vi "ConvertControlTerminals.vi"(5 "PythonConverter_BD in":refnum<class "PyConvBD.lvclass">, 6 "error in":errorcluster, 9 "Diagram in":refnum<class "Diagram.lvclass">) -> (0 "error out":errorcluster, 3 "Diagram out":refnum<class "Diagram.lvclass">, 4 "PythonConverter_BD out":refnum<class "PyConvBD.lvclass">)   [LabVIEW 2014, in "Raspberry Pi Compatible Compiler for LabVIEW.lvlib" / "Diagram.lvclass"]
uses:
  Diagram.lvclass
  Python/PythonConverter_BD/PyConvBD.lvclass
  Terminal/Terminal.lvclass
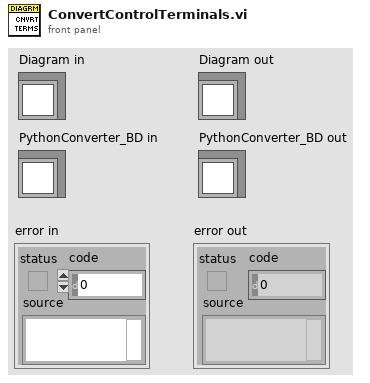
[diagram p1: front panel]
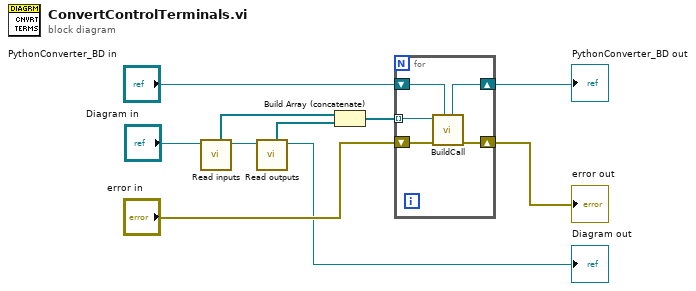
[diagram p0: block diagram]
diagram:
  n1 = call-dynamic "Read inputs.vi"("Diagram in"="Diagram in") -> ("Diagram out"=w9:refnum<class "Diagram.lvclass">, "inputs"=w8:refnum<class "Terminal.lvclass">[])  [unwired: 7 in]
  n2 = call-dynamic "Read outputs.vi"("Diagram in"=w9) -> ("Diagram out"=→"Diagram out":refnum<class "Diagram.lvclass">, "outputs"=w7:refnum<class "Terminal.lvclass">[])  [unwired: 7 in]
  n3 = Build Array (concatenate)(w8, w7) -> (w6:refnum<class "Terminal.lvclass">[])
  n4 = for {
    tunnel: w6 -> [w11] mode=indexing
    shift-right: [w14] -> w3
    shift-left: "PythonConverter_BD in" -> [w15]
    shift-right: [w12] -> w2
    shift-left: "error in" -> [w13]
    n5 = call-dynamic "BuildCall.vi"("PythonConverter_BD in"=w15, "error in"=w13, "Terminal in"=w11) -> ("error out"=w12:errorcluster, "PythonConverter_BD out"=w14:refnum<class "PyConvBD.lvclass">)  [unwired: 6 in, 1 out]
  }
  "error out" <- w2
  "PythonConverter_BD out" <- w3
